vi "FPGA-7842R-Control V1.vi"(0 "Waveform Data":T4, 2 "Action":T5=enum."Exit", 3 "Laser On Time (Ticks)":u8=13, 5 "Laser Controls":T1 {"STED Power (V)" scale=0.0..10.0}, 7 "Manual Controls":T3={"Galvo 1 Position (I16)"=-280, "Galvo 2 Position (I16)"=-280, "X Axis Voltage (I16)"=0, "Y Axis Voltage (I16)"=0, "Z Axis Voltage (I16)"=0, "Res Mirror Amp (I16)"=0, "Res Mirror Mute"=FALSE, "Upper Shutter"=FALSE, "Lower Shutter"=FALSE}, 9 "Image Acquisition Parameters":T2={"Scan Type"=enum."Sample Scanning", "Scan Mode"=enum."XY", "Fast Axis Frequency (Hz)"=100.0, "Image Format"=128, "Line Accumulations"=1, "Frames Per Capture"=1, "Frames Accumulations"=1, "Image Dimension (um)"=[], "Number of Z Steps"=1, "Z Steps Size (um)"=1.0, "Pixel Size (nm)"=[]} {"Z Steps Size (um)" min=0.0; "Number of Z Steps" min=1; "Frames Accumulations" min=1; "Frames Per Capture" min=1; "Line Accumulations" min=1; "Image Format" items=["64 x 64"=64, "128 x 128"=128, "256 x 256"=256, "512 x 512"=512, "1024 x 1024"=1024, "2048 x 2048"=2048]}, 11 "Initialize":bool, 12 "Unused Axis Offset (I16)":i16, 14 "Laser Delay (Ticks)":u8=6) -> (4 "Shutter Status":cluster{"US Status":bool, "LS Status":bool}, 15 "Initalized":bool)   [LabVIEW 2014]
uses:
  FPGA-7842R-Reference.ctl
  Waveform Data.ctl
  Manual Controls V2.ctl
  Type Defs/Image Acquisition Parameters.ctl
  Laser Controls.ctl
  <vilib>/FPGAPlugInAG/PCIe-7841R/niLvFpga_Open_PCIe-7841R.vi
  <vilib>/Utility/error.llb/Error Cluster From Error Code.vi
  <vilib>/rvi/errors/niLvFpgaAdjustHostInterfaceError.vi
  <vilib>/FPGAPlugInAG/PCIe-7841R/niLvFpga_Run_PCIe-7841R.vi
  <vilib>/FPGAPlugInAG/PCIe-7841R/niLvFpga_Close_PCIe-7841R.vi
  <vilib>/rvi/interface/nirviOpenFPGA/nirviOpenFPGA.xnode
  FPGA Bitfiles/MainSTEDFPGAProj_FPGATarget_WaveformandLaser_ZYWKw02D2jI.lvbitx
  FPGA Target VIs/FPGA-7841R/Waveform and Laser Controls V5.vi
  <vilib>/rvi/interface/nirviReadWriteControl/nirviReadWriteControl.xnode
  FPGA Target VIs/FPGA-7841R/Waveform Scan Parameters.ctl
  <vilib>/rvi/interface/nirviMethod/nirviMethod.xnode
  <vilib>/rvi/interface/nirviCloseFPGA/nirviCloseFPGA.xnode
  NiFpgaLv.dll
panel:
  # "XY"
  # "Z"
  # "Length"
  # "Height"
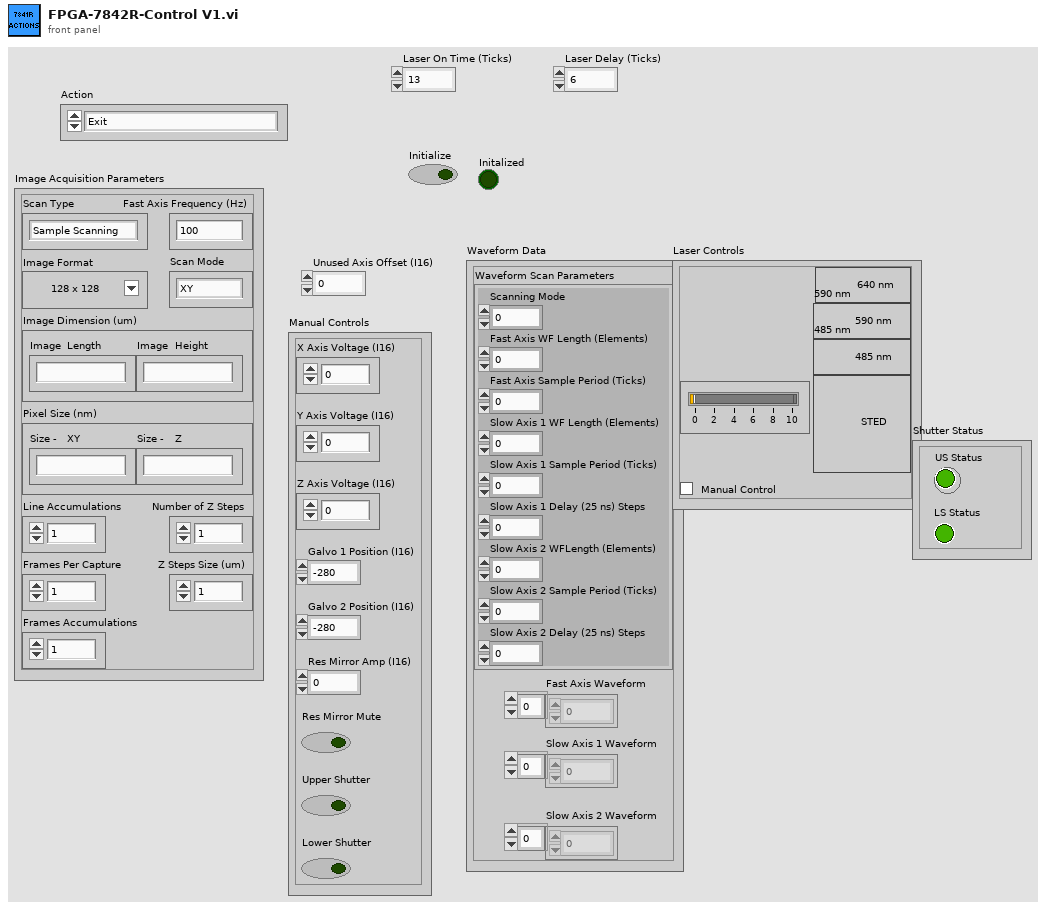
[diagram p1: front panel]
types:
  T1 = typedef "Laser Controls.ctl" = cluster{"STED Power (V)":dbl, "STED":bool, "650 nm":bool, "590 nm":bool, "485 nm":bool, "Manual Control":bool}
  T2 = typedef "Image Acquisition Parameters.ctl" = cluster{"Scan Type":enum16{"Sample Scanning", "Beam Scanning"}, "Scan Mode":enum16{"XY", "XZ", "YZ", "XYZ"}, "Fast Axis Frequency (Hz)":dbl, "Image Format":u16, "Line Accumulations":u16, "Frames Per Capture":u16, "Frames Accumulations":u16, "Image Dimension (um)":dbl[], "Number of Z Steps":u8, "Z Steps Size (um)":dbl, "Pixel Size (nm)":dbl[]}
  T3 = typedef "Manual Controls V2.ctl" = cluster{"Galvo 1 Position (I16)":i16, "Galvo 2 Position (I16)":i16, "X Axis Voltage (I16)":i16, "Y Axis Voltage (I16)":i16, "Z Axis Voltage (I16)":i16, "Res Mirror Amp (I16)":i16, "Res Mirror Mute":bool, "Upper Shutter":bool, "Lower Shutter":bool}
  T4 = typedef "Waveform Data.ctl" = cluster{"Waveform Scan Parameters":cluster{"Scanning Mode":u8, "Fast Axis WF Length (Elements)":i32, "Fast Axis Sample Period (Ticks)":u32, "Slow Axis 1 WF Length (Elements)":i32, "Slow Axis 1 Sample Period (Ticks)":u32, "Slow Axis 1 Delay (25 ns) Steps":i32, "Slow Axis 2 WFLength (Elements)":i32, "Slow Axis 2 Sample Period (Ticks)":u32, "Slow Axis 2 Delay (25 ns) Steps":i32}, "Fast Axis Waveform":dbl[], "Slow Axis 1 Waveform":dbl[], "Slow Axis 2 Waveform":dbl[]}
  T5 = typedef "FPGA-7842R-Reference.ctl" = enum16{"Stage Control", "Laser Control", "Unused Axis I16", "Exit", "Set Res Mirror", "Set Galvo", "Current Frame for Capture", "Default", "Close FPGA", "Stop Waveforms", "Start Waveforms", "Shutter Control", "Initialize"}
  T6 = cluster{"Scanning Mode":u8, "Fast Axis WF Length (Elements)":i32, "Fast Axis Sample Period (Ticks)":u32, "Slow Axis 1 WF Length (Elements)":i32, "Slow Axis 1 Sample Period (Ticks)":u32, "Slow Axis 1 Delay (25 ns) Steps":i32, "Slow Axis 2 WFLength (Elements)":i32, "Slow Axis 2 Sample Period (Ticks)":u32, "Slow Axis 2 Delay (25 ns) Steps":i32}
  T7 = cluster{"Res Mirror Amp (I16)":i16, "Res Mirror Mute":bool}
  T8 = typedef "Scan Parameters.ctl" = cluster{"Fast_Ax_Amp_V":dbl, "Fast_Ax_Off_V":dbl, "Slow_Ax_Amp_V":dbl, "Slow_Ax_Off_V ":dbl, "Slow_Ax_Max_V_VperS":dbl, "Slow_Ax1_Del25ns":i32, "Slow_Ax2_Del25ns":i32, "Stage_X_Off_V":dbl, "Stage_Y_Off_V":dbl, "Stage_Z_Off_V":dbl, "Galvo1_Off_V":dbl, "Galvo2_Off_V":dbl, "Last_Scan_Mode":enum16{"XY", "XZ", "YZ", "XYZ"}, "Current_Scan_Mode":enum16{"XY", "XZ", "YZ", "XYZ"}, "Fly_Back_Lines":u16, "Linear_Ramp_End":u32, "Z_Step_I16":i16, "Z_Start_I16":i16, "Laser_States _U32":u32, "590_Voltage_I16":i16, "775_AOM_Volt_I16":i16, "Blanking OFF":bool, "Unused_Axis_I16":i16}
  T9 = cluster{"Upper Shutter Status":bool, "Lower Shutter Status":bool}
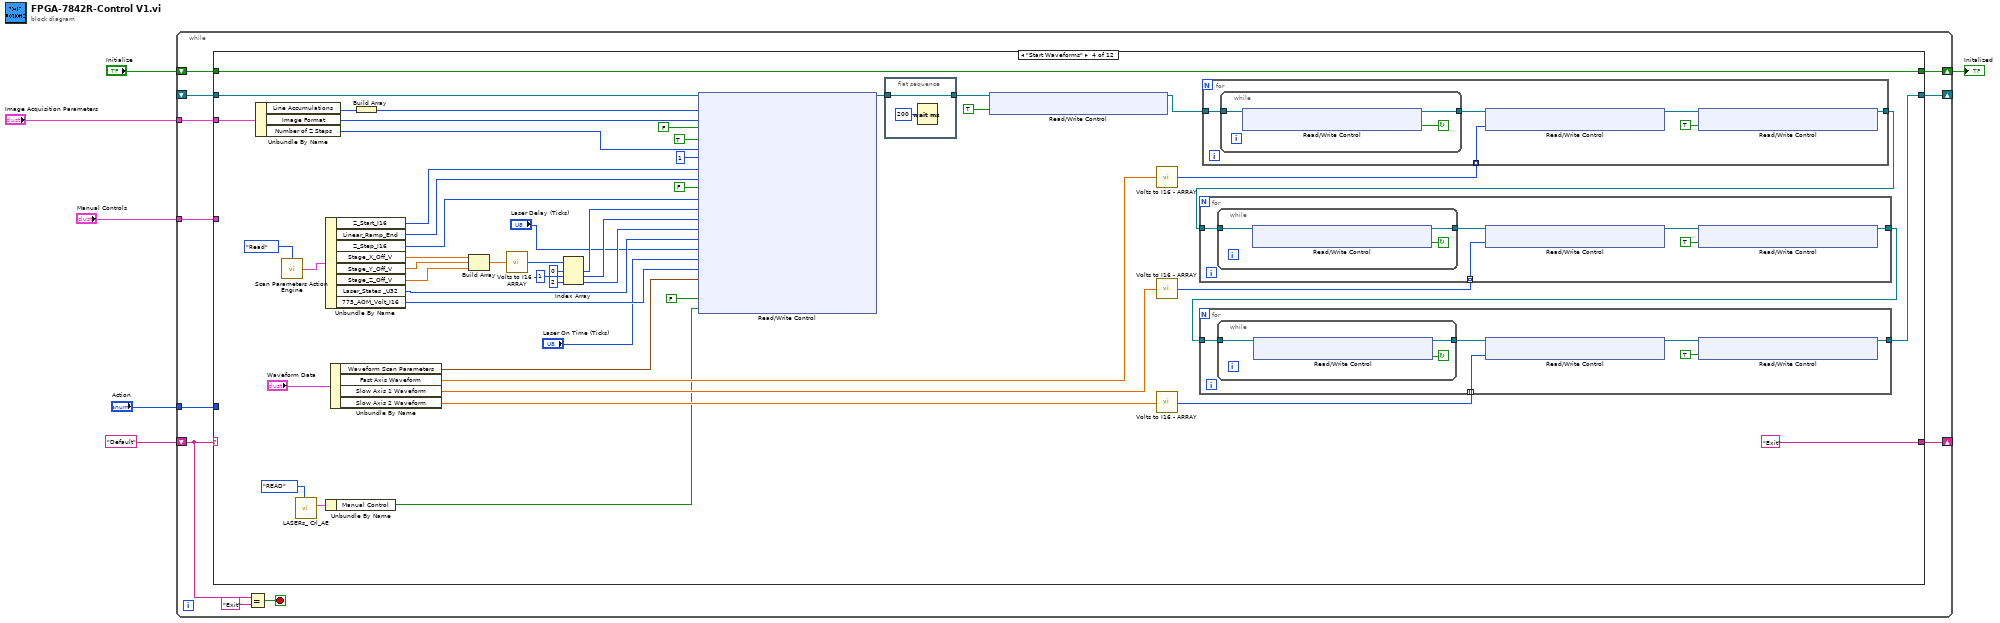
[diagram p0: block diagram]
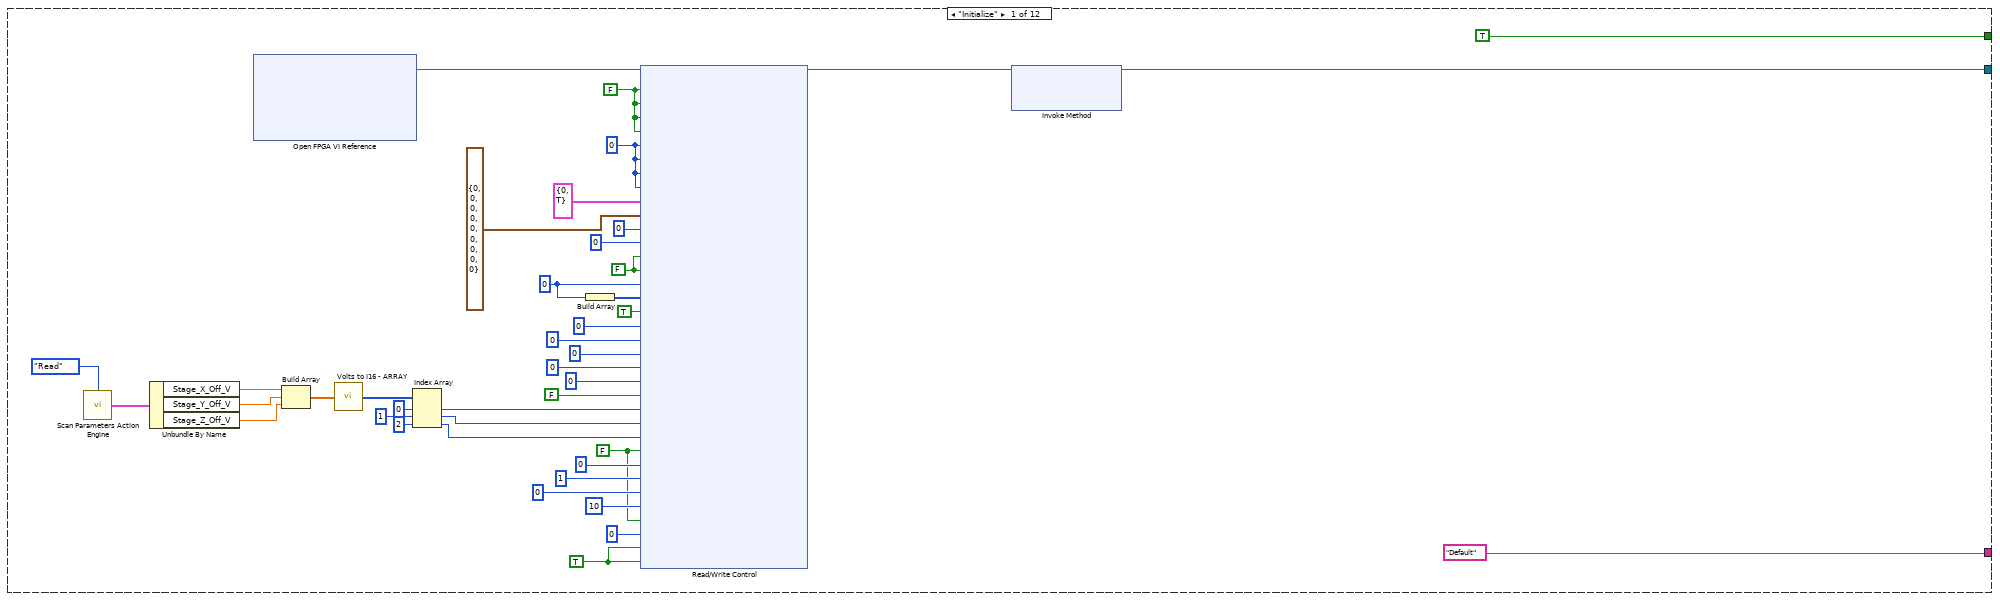
[diagram p2: hidden frame]
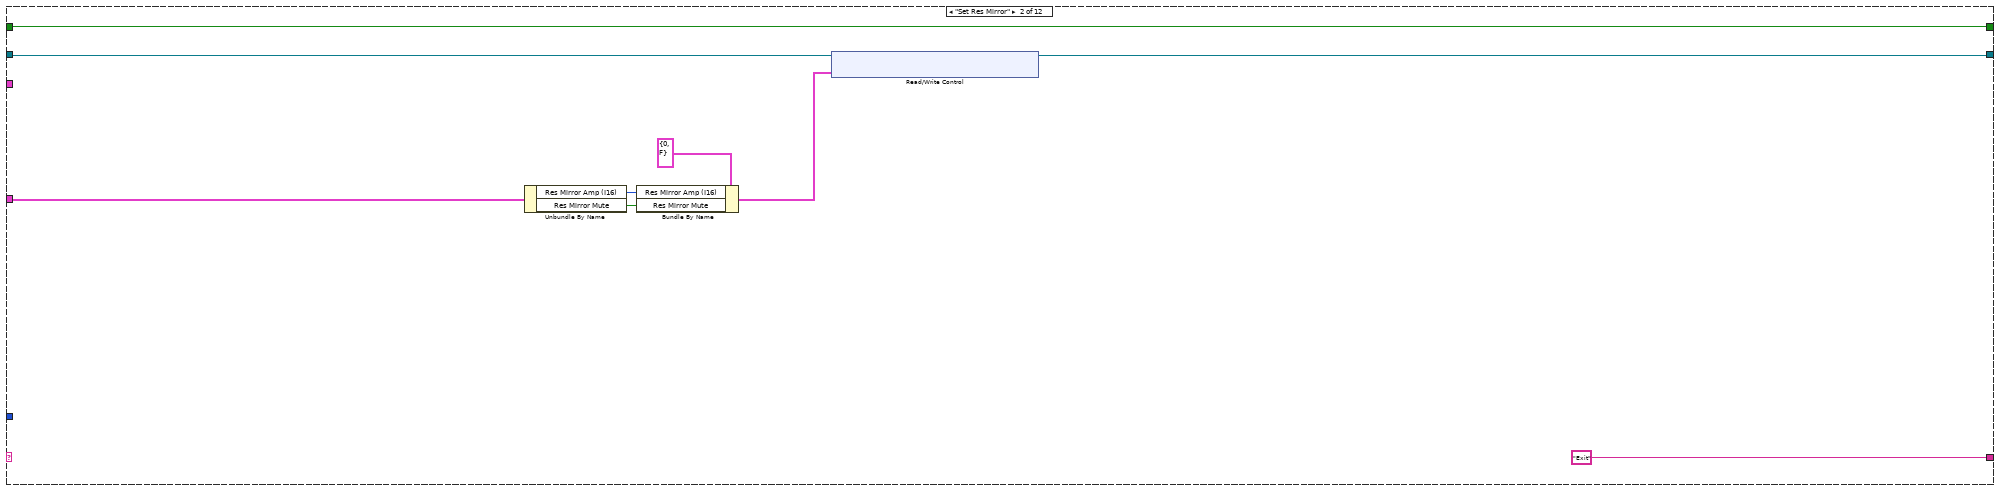
[diagram p3: hidden frame]
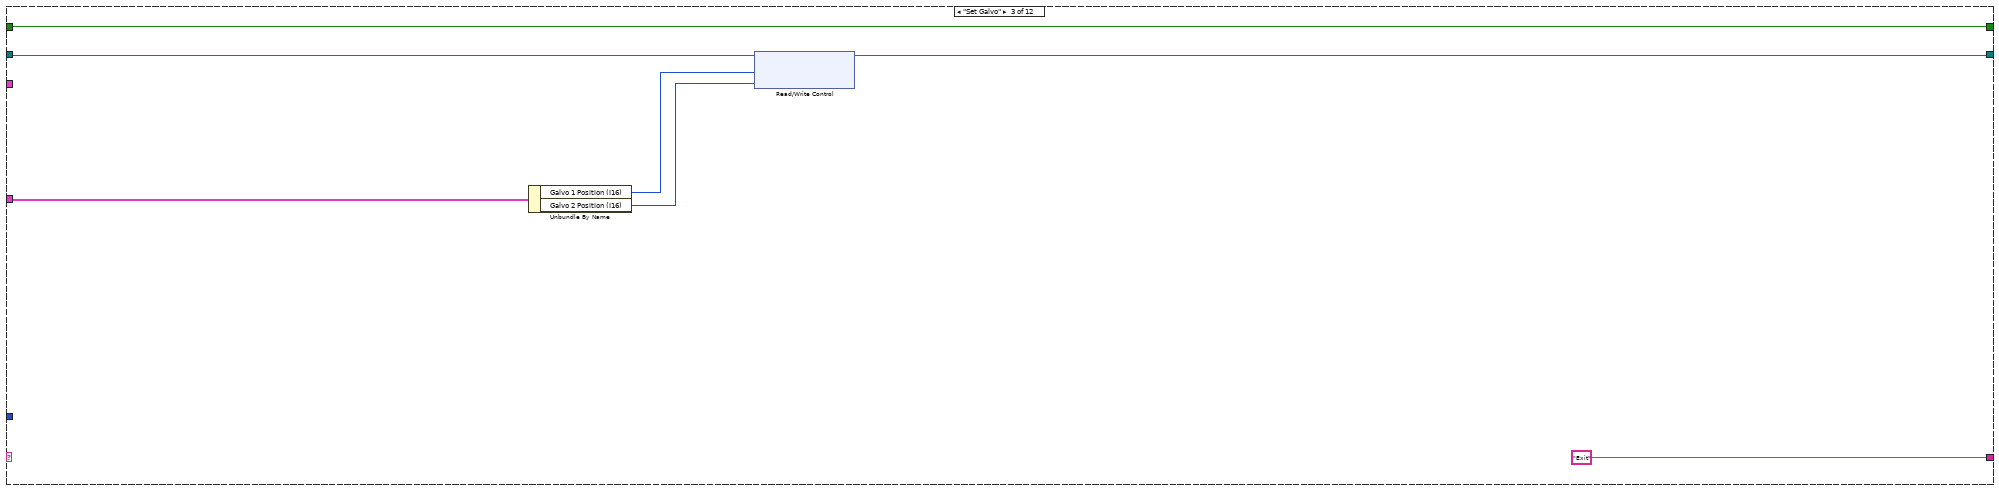
[diagram p4: hidden frame]
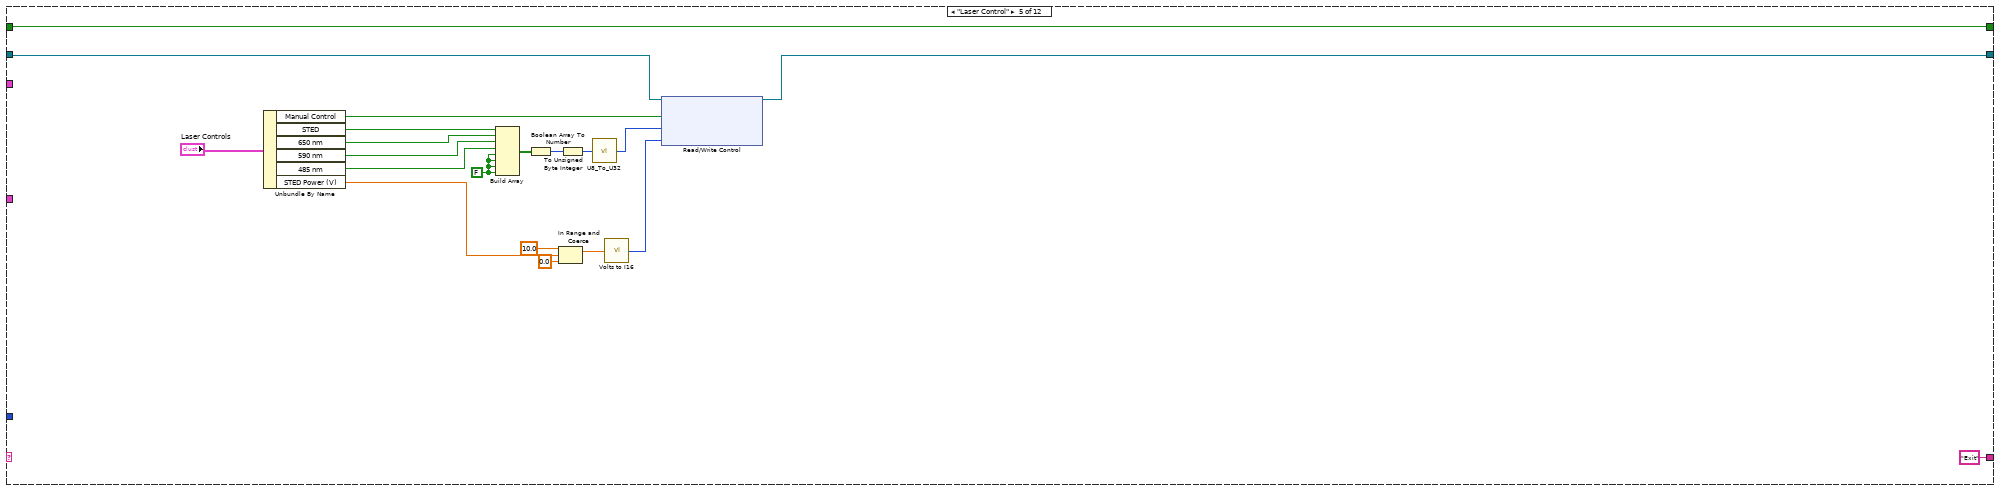
[diagram p5: hidden frame]
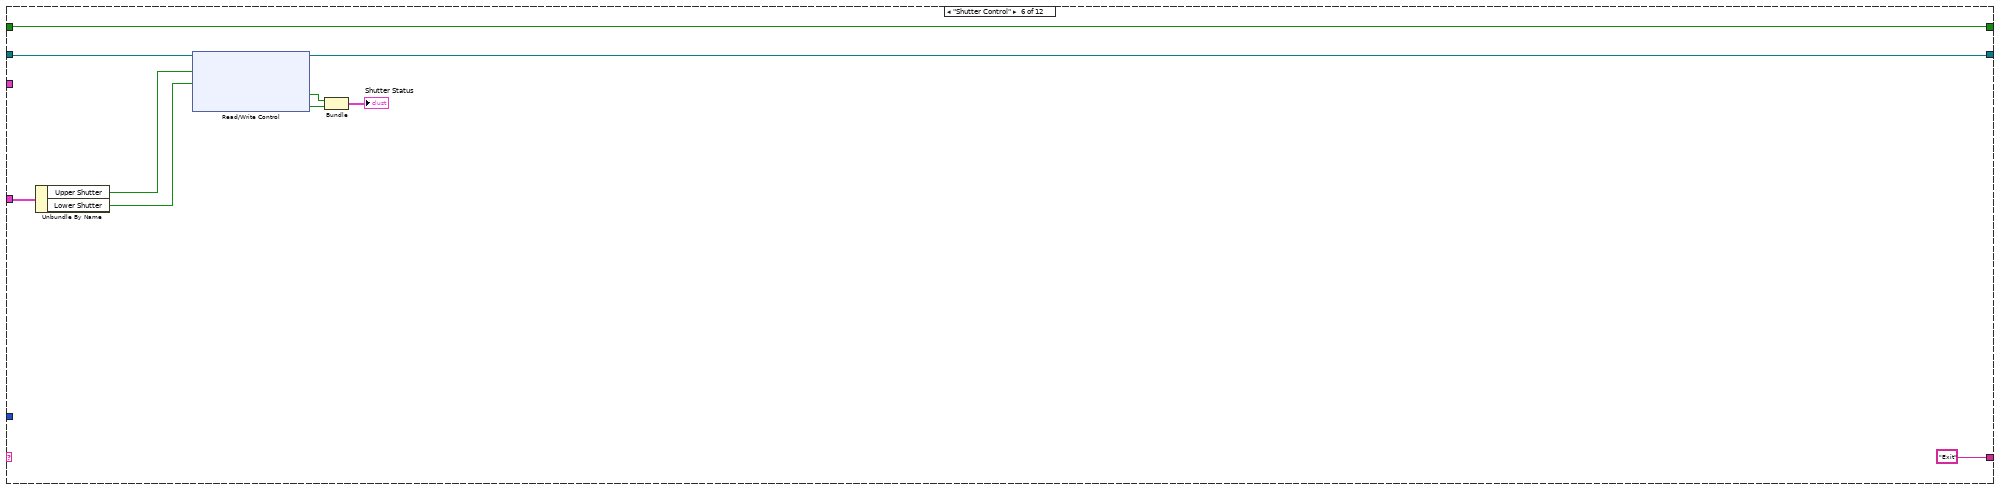
[diagram p6: hidden frame]
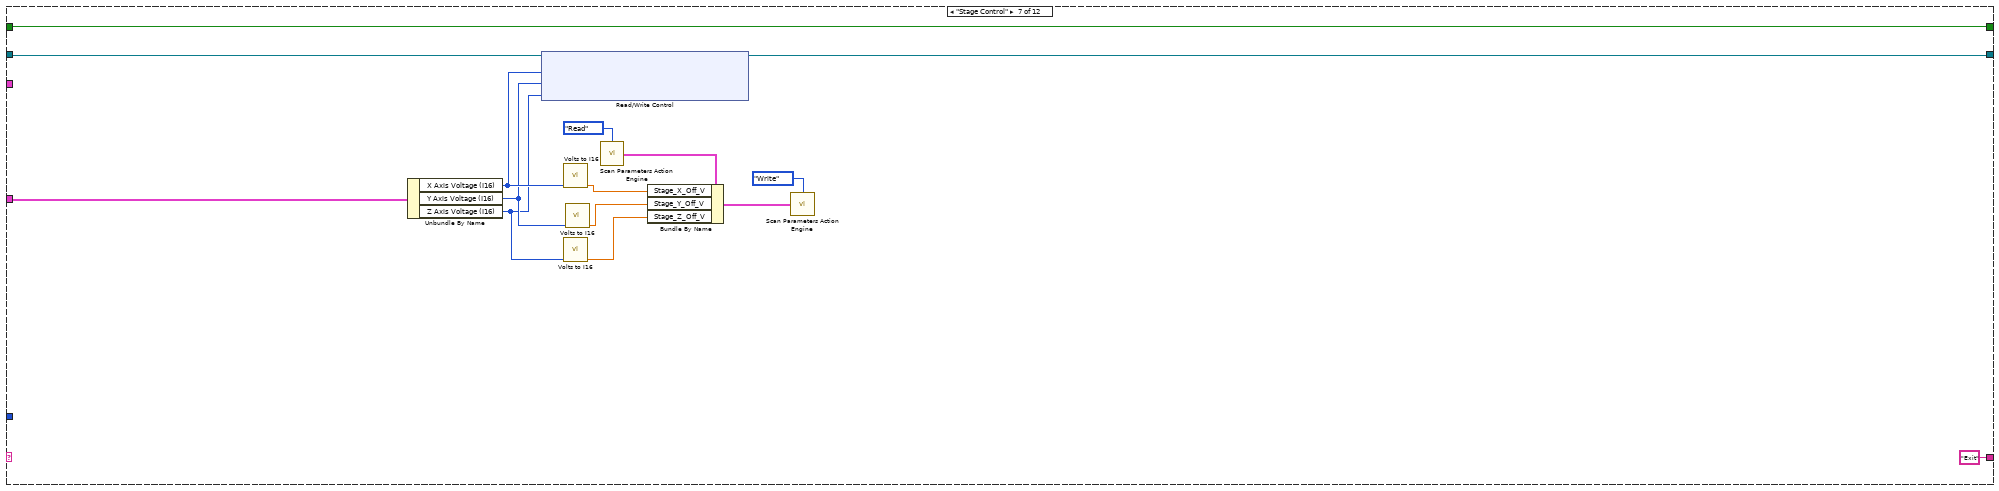
[diagram p7: hidden frame]
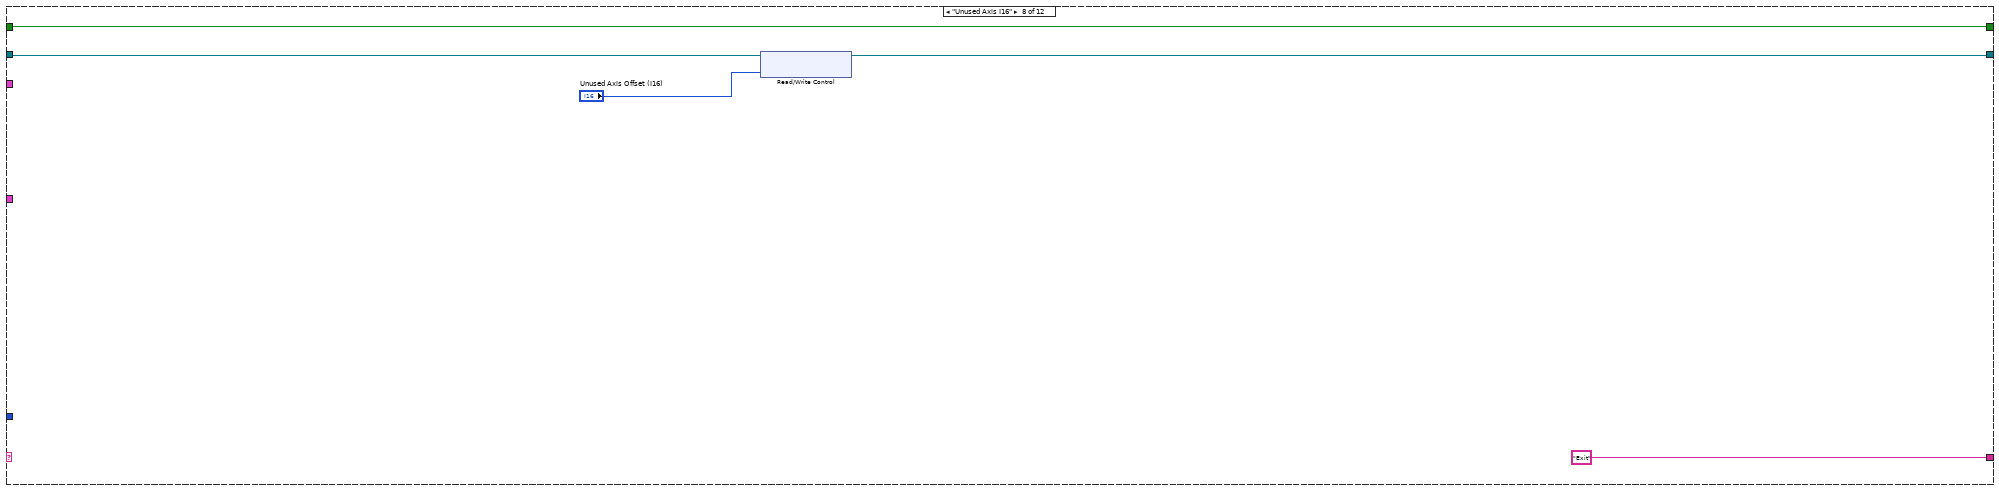
[diagram p8: hidden frame]
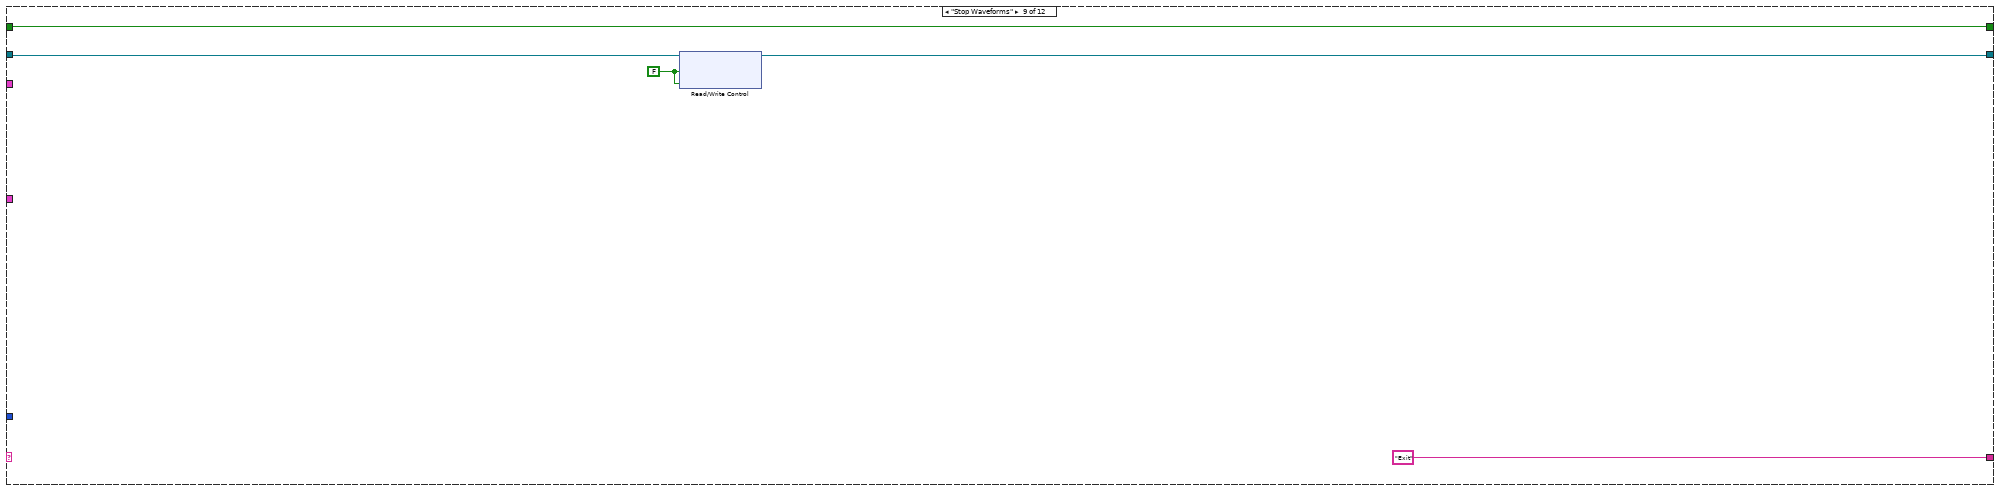
[diagram p9: hidden frame]
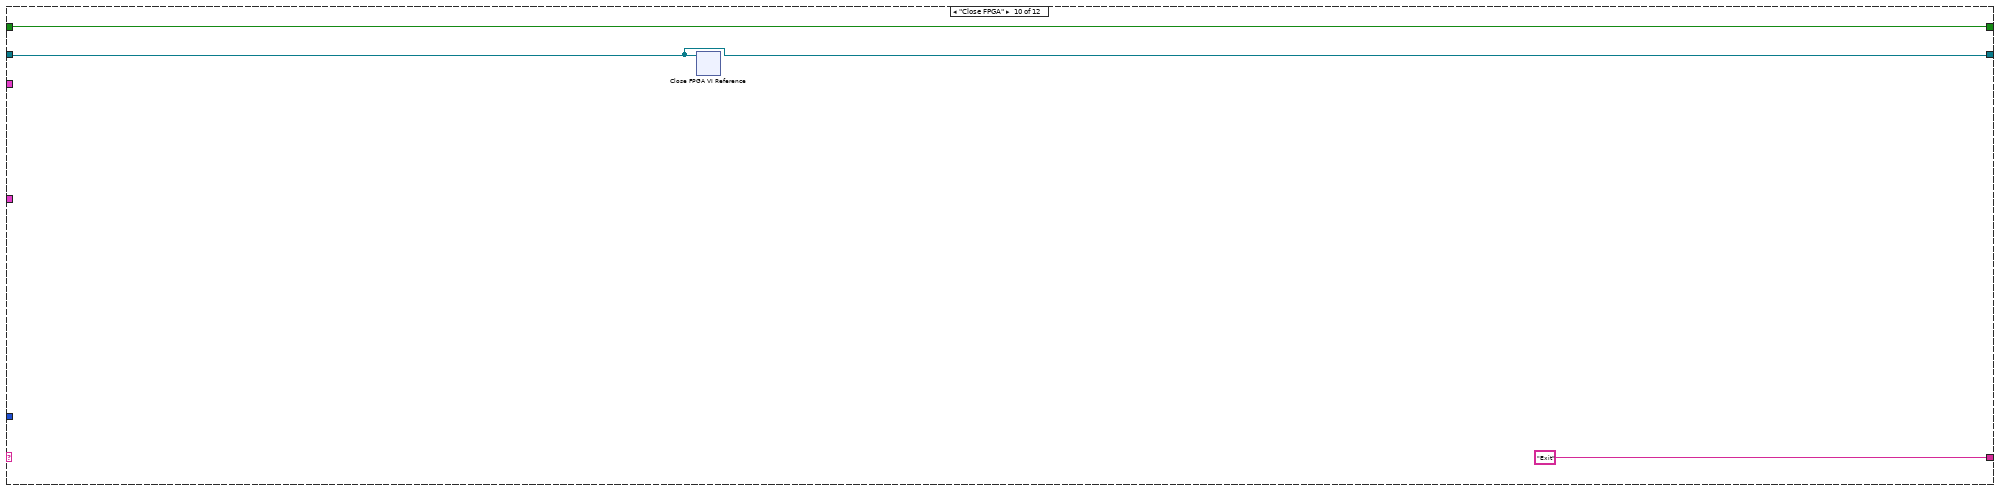
[diagram p10: hidden frame]
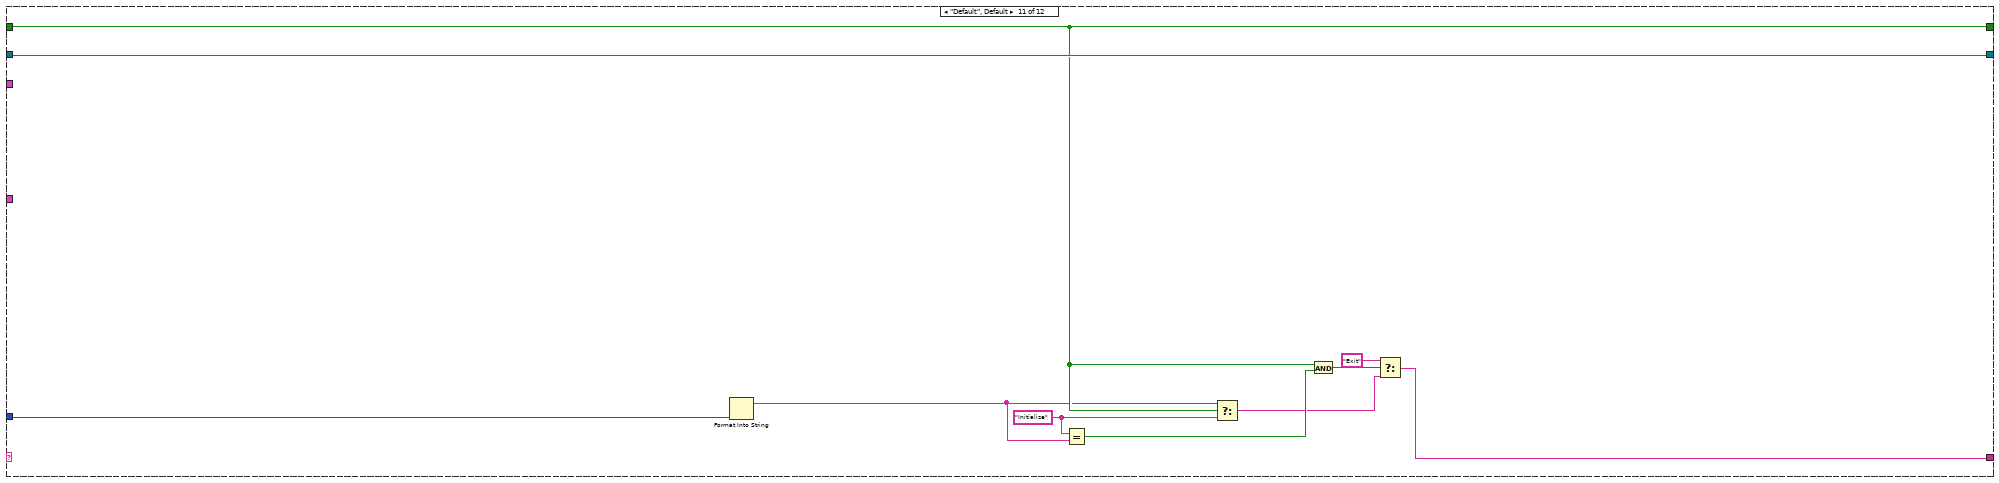
[diagram p11: hidden frame]
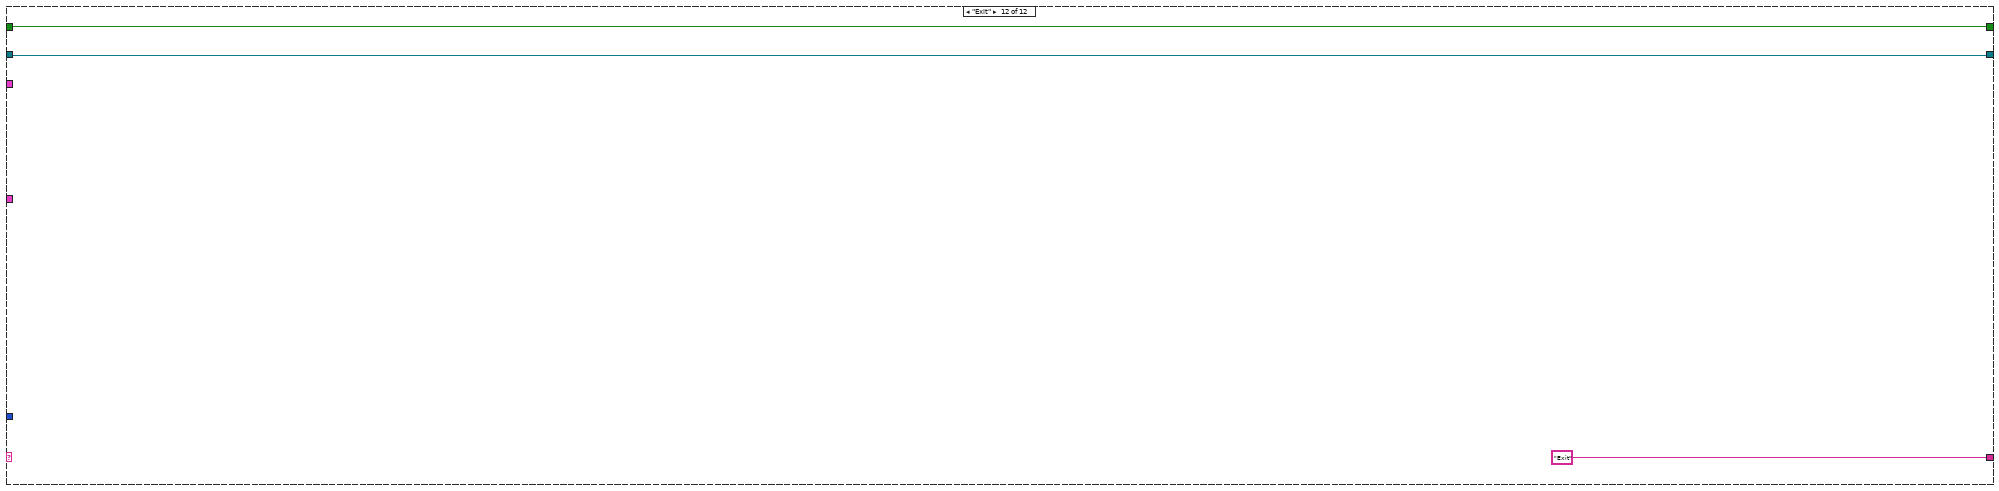
[diagram p12: hidden frame]
diagram:
  n1 = while {
    shift-right: [w17] -> _
    shift-left: _ -> [w16]
    shift-right: [w14] -> _
    shift-left: "Default" -> [w13]
    tunnel: "Action" -> [w15]
    shift-right: [w10] -> w3
    shift-left: "Initialize" -> [w9]
    tunnel: "Manual Controls" -> [w8]
    tunnel: "Image Acquisition Parameters" -> [w7]
    stop <- w11 stop-if-true
    n2 = case shown="\"Start Waveforms\"" w13 {
      tunnel: [w49 w64 w71 w114 w170 w182 w195 w201 w208 w210 w222 w224] -> w17
      tunnel: w16 -> [_ w65 w72 w117 w171 w183 w196 w202 w209 w210 w222 w224]
      tunnel: w15 -> [_ _ _ _ _ _ _ _ _ _ w221 _]
      tunnel: ["Default" ("f") "Exit" ("f") "Exit" ("f") "Exit" ("f") "Exit" ("f") "Exit" ("f") "Exit" ("f") "Exit" ("f") "Exit" ("f") "Exit" ("f") w215 "Exit" ("f")] -> w14
      tunnel: [TRUE w67 w74 w119 w173 w184 w198 w204 w207 w212 w220 w225] -> w10
      tunnel: w9 -> [_ w67 w74 w119 w173 w184 w198 w204 w207 w212 w220 w225]
      tunnel: w8 -> [_ w63 w70 _ _ w177 w197 _ _ _ _ _]
      tunnel: w7 -> [_ _ _ w108 _ _ _ _ _ _ _ _]
      frame "Initialize" {
        w18 = TRUE ("Upper Shutter Command")
        w20 = FALSE ("Blanking Off/Manual")
        w45 = u16 0 ("Number of Lines")
        w47 = FALSE ("Reset Position Error")
        w58 = i16 0 ("Fast Axis Waveform Element")
        w57 = FALSE ("WF 1 Data Loaded")
        n3 = call "Scan Parameters Action Engine.vi"("Action"=enum16{"Read", "Write"}."Read") -> ("Scan Parameters OUT"=w36:T8)  [unwired: 14 in]
        n4 = Unbundle By Name(w36) -> ("Stage_X_Off_V"=w35:dbl, "Stage_Y_Off_V"=w33:dbl, "Stage_Z_Off_V"=w34:dbl)
        n5 = xnode "Open FPGA VI Reference"() -> ("FPGA VI Reference Out"=w48:refnum<k20>)  [unwired: 2 in, 1 out]
        n6 = Build Array(w35, w33, w34) -> (w32:dbl[])
        n7 = call "Volts to I16 - ARRAY.vi"("Voltage (V)"=w32) -> ("I16"=w31:i16[])  [unwired: 14 in]
        n8 = Index Array(array=w31, index #1=0 ("index"), index #2=1 ("index"), index #3=2 ("index")) -> (element #1=w27:i16, element #2=w25:i16, element #3=w26:i16)
        n9 = Build Array(w45) -> (w44:u16[])
        n10 = xnode "Read/Write Control"("FPGA VI Reference In"=w48, "WF 1 Data Loaded"=w57, "WF 2 Data Loaded"=w57, "WF 3 Data Loaded"=w57, "Start Waveforms"=w57, "Fast Axis Waveform Element"=w58, "Slow Axis 1 Waveform Element"=w58, "Slow Axis 2 Waveform Element"=w58, "Unused Axis Offset"=w58, "Resonant Mirror"=T7 {"Res Mirror Amp (I16)"=0, "Res Mirror Mute"=TRUE} ("Resoance Mirror"), "Waveform Scan Parameters"=T6 {"Scanning Mode"=0, "Fast Axis WF Length (Elements)"=0, "Fast Axis Sample Period (Ticks)"=0, "Slow Axis 1 WF Length (Elements)"=0, "Slow Axis 1 Sample Period (Ticks)"=0, "Slow Axis 1 Delay (25 ns) Steps"=0, "Slow Axis 2 WFLength (Elements)"=0, "Slow Axis 2 Sample Period (Ticks)"=0, "Slow Axis 2 Delay (25 ns) Steps"=0}, "Galvo 2 Position (I16)"=i16 0, "Galvo 1 Position (I16)"=i16 0, "Reset Position Error"=w47, "Frame Trigger"=w47, "Number of Lines"=w45, "Accums Per Line"=w44, "Stop Sync Signal"=TRUE, "Z Step Size (I16)"=i16 0, "Number of Z Steps"=u8 0, "Frames Per Z Step"=u8 0, "Z Stack Start Position (I16)"=i16 0, "End of Linear Ramp"=u32 0, "End Linear Ramp"=FALSE, "X Piezo Axis"=w27, "Y Piezo Axis"=w25, "Z Piezo Axis"=w26, "Blanking Off/Manual"=w20, "Laser States"=u32 0, "Laser Delay (Ticks)"=u8 1, "Sequences"=u8 0, "Laser On Time (Ticks)"=u8 10, "Laser Blank Trigger"=w20, "775 AOM (I16)"=i16 0 ("590 Analog Voltage (I16)"), "Upper Shutter Command"=w18, "Lower Shutter Command"=w18) -> ("FPGA VI Reference Out"=w54:refnum<k20>)  [unwired: 1 in, 1 out]
        n11 = xnode "Invoke Method"("FPGA VI Reference In"=w54) -> ("FPGA VI Reference Out"=w49:refnum<k20>)  [unwired: 2 in, 1 out]
      }
      frame "Set Res Mirror" {
        n12 = Unbundle By Name(w63) -> ("Res Mirror Amp (I16)"=w62:i16, "Res Mirror Mute"=w61:bool)
        n13 = Bundle By Name(cluster=T7 {"Res Mirror Amp (I16)"=0, "Res Mirror Mute"=FALSE} ("Resoance Mirror"), "Res Mirror Amp (I16)"=w62, "Res Mirror Mute"=w61) -> (w59:T7)
        n14 = xnode "Read/Write Control"("FPGA VI Reference In"=w65, "Resonant Mirror"=w59) -> ("FPGA VI Reference Out"=w64:refnum<k20>)  [unwired: 1 in, 1 out]
      }
      frame "Set Galvo" {
        n15 = Unbundle By Name(w70) -> ("Galvo 1 Position (I16)"=w69:i16, "Galvo 2 Position (I16)"=w68:i16)
        n16 = xnode "Read/Write Control"("FPGA VI Reference In"=w72, "Galvo 1 Position (I16)"=w69, "Galvo 2 Position (I16)"=w68) -> ("FPGA VI Reference Out"=w71:refnum<k20>)  [unwired: 1 in, 1 out]
      }
      frame "Start Waveforms" {
        n17 = Unbundle By Name(w108) -> ("Line Accumulations"=w106:u16, "Image Format"=w107:u16, "Number of Z Steps"=w97:u8)
        n18 = call "Scan Parameters Action Engine.vi"("Action"=enum16{"Read", "Write"}."Read") -> ("Scan Parameters OUT"=w101:T8)  [unwired: 14 in]
        n19 = call "LASERs_ Crl_AE.vi"("Action"=enum16{"READ", "WRITE"}."READ") -> ("Detectors Parameters Out"=w76:T1)  [unwired: 10 in]
        n20 = Unbundle By Name(w101) -> ("Z_Start_I16"=w99:i16, "Linear_Ramp_End"=w100:u32, "Z_Step_I16"=w96:i16, "Stage_X_Off_V"=w89:dbl, "Stage_Y_Off_V"=w88:dbl, "Stage_Z_Off_V"=w87:dbl, "Laser_States _U32"=w83:u32, "775_AOM_Volt_I16"=w82:i16)
        n21 = Unbundle By Name(w76) -> ("Manual Control"=w75:bool)
        n22 = Unbundle By Name("Waveform Data") -> ("Waveform Scan Parameters"=w81:T6, "Fast Axis Waveform"=w121:dbl[], "Slow Axis 1 Waveform"=w113:dbl[], "Slow Axis 2 Waveform"=w120:dbl[])
        n23 = Build Array(w106) -> (w105:u16[])
        n24 = Build Array(w89, w88, w87) -> (w94:dbl[])
        n25 = call "Volts to I16 - ARRAY.vi"("Voltage (V)"=w94) -> ("I16"=w93:i16[])  [unwired: 14 in]
        n26 = Index Array(array=w93, index #1=0 ("index"), index #2=1 ("index"), index #3=2 ("index")) -> (element #1=w86:i16, element #2=w85:i16, element #3=w84:i16)
        n27 = xnode "Read/Write Control"("FPGA VI Reference In"=w117, "Accums Per Line"=w105, "Number of Lines"=w107, "Frame Trigger"=FALSE, "Stop Sync Signal"=TRUE, "Number of Z Steps"=w97, "Frames Per Z Step"=u8 1, "Z Stack Start Position (I16)"=w99, "End of Linear Ramp"=w100, "End Linear Ramp"=FALSE, "Z Step Size (I16)"=w96, "X Piezo Axis"=w86, "Y Piezo Axis"=w85, "Z Piezo Axis"=w84, "Laser States"=w83, "Laser Delay (Ticks)"="Laser Delay (Ticks)", "Laser On Time (Ticks)"="Laser On Time (Ticks)", "775 AOM (I16)"=w82, "Waveform Scan Parameters"=w81, "Frame Trigger"=FALSE, "Blanking Off/Manual"=w75) -> ("FPGA VI Reference Out"=w115:refnum<k20>)  [unwired: 1 in, 2 out]
        n28 = flat-sequence {
          tunnel: [w127] -> w116
          tunnel: w115 -> [w127]
          frame #0 {
            n29 = Wait (ms)(milliseconds to wait=u32 200) -> ()  [unwired: 1 out]
          }
        }
        n30 = xnode "Read/Write Control"("FPGA VI Reference In"=w116, "Start Waveforms"=TRUE) -> ("FPGA VI Reference Out"=w122:refnum<k20>)  [unwired: 1 in, 1 out]
        n31 = call "Volts to I16 - ARRAY.vi"("Voltage (V)"=w121) -> ("I16"=w125:i16[])  [unwired: 14 in]
        n32 = call "Volts to I16 - ARRAY.vi"("Voltage (V)"=w113) -> ("I16"=w111:i16[])  [unwired: 14 in]
        n33 = call "Volts to I16 - ARRAY.vi"("Voltage (V)"=w120) -> ("I16"=w112:i16[])  [unwired: 14 in]
        n34 = for {
          tunnel: w122 -> [w150]
          tunnel: [w148] -> w124
          tunnel: w125 -> [w146] mode=indexing
          n35 = while {
            tunnel: w150 -> [w154]
            tunnel: [w153] -> w149
            stop <- w152 continue-if-true
            n36 = xnode "Read/Write Control"("FPGA VI Reference In"=w154) -> ("FPGA VI Reference Out"=w153:refnum<k20>, "WF 1 Data Loaded"=w152:bool)  [unwired: 1 in, 1 out]
          }
          n37 = xnode "Read/Write Control"("FPGA VI Reference In"=w149, "Fast Axis Waveform Element"=w146) -> ("FPGA VI Reference Out"=w151:refnum<k20>)  [unwired: 1 in, 1 out]
          n38 = xnode "Read/Write Control"("FPGA VI Reference In"=w151, "WF 1 Data Loaded"=TRUE ("Host Data Loaded")) -> ("FPGA VI Reference Out"=w148:refnum<k20>)  [unwired: 1 in, 1 out]
        }
        n39 = for {
          tunnel: w124 -> [w141]
          tunnel: [w139] -> w95
          tunnel: w111 -> [w137] mode=indexing
          n40 = while {
            tunnel: w141 -> [w145]
            tunnel: [w144] -> w140
            stop <- w143 continue-if-true
            n41 = xnode "Read/Write Control"("FPGA VI Reference In"=w145) -> ("FPGA VI Reference Out"=w144:refnum<k20>, "WF 2 Data Loaded"=w143:bool)  [unwired: 1 in, 1 out]
          }
          n42 = xnode "Read/Write Control"("FPGA VI Reference In"=w140, "Slow Axis 1 Waveform Element"=w137) -> ("FPGA VI Reference Out"=w142:refnum<k20>)  [unwired: 1 in, 1 out]
          n43 = xnode "Read/Write Control"("FPGA VI Reference In"=w142, "WF 2 Data Loaded"=TRUE ("Host Data Loaded")) -> ("FPGA VI Reference Out"=w139:refnum<k20>)  [unwired: 1 in, 1 out]
        }
        n44 = for {
          tunnel: w95 -> [w132]
          tunnel: [w130] -> w114
          tunnel: w112 -> [w128] mode=indexing
          n45 = while {
            tunnel: w132 -> [w136]
            tunnel: [w135] -> w131
            stop <- w134 continue-if-true
            n46 = xnode "Read/Write Control"("FPGA VI Reference In"=w136) -> ("FPGA VI Reference Out"=w135:refnum<k20>, "WF 3 Data Loaded"=w134:bool)  [unwired: 1 in, 1 out]
          }
          n47 = xnode "Read/Write Control"("FPGA VI Reference In"=w131, "Slow Axis 2 Waveform Element"=w128) -> ("FPGA VI Reference Out"=w133:refnum<k20>)  [unwired: 1 in, 1 out]
          n48 = xnode "Read/Write Control"("FPGA VI Reference In"=w133, "WF 3 Data Loaded"=TRUE ("Host Data Loaded")) -> ("FPGA VI Reference Out"=w130:refnum<k20>)  [unwired: 1 in, 1 out]
        }
      }
      frame "Laser Control" {
        w164 = FALSE ("element")
        n49 = Unbundle By Name("Laser Controls") -> ("Manual Control"=w172:bool, "STED"=w161:bool, "650 nm"=w160:bool, "590 nm"=w159:bool, "485 nm"=w158:bool, "STED Power (V)"=w157:dbl)
        n50 = Build Array(w161, w160, w159, w158, w164, w164, w164, w164) -> (w162:bool[])
        n51 = Boolean Array To Number(Boolean array=w162) -> (number=w163:u32)
        n52 = In Range and Coerce(upper limit=10.0, x=w157, lower limit=0.0) -> (coerced(x)=w168:dbl)  [unwired: 1 out]
        n53 = To Unsigned Byte Integer(number=w163) -> (unsigned 8bit integer=w165:u8)
        n54 = call "U8_To_U32.vi"("U8 IN"=w165) -> ("U32 OUT"=w156:u32)  [unwired: 13 in, 1 out]
        n55 = call "Volts to I16.vi"("Voltage (V)"=w168) -> ("I16"=w155:i16)  [unwired: 13 in, 1 out]
        n56 = xnode "Read/Write Control"("FPGA VI Reference In"=w171, "Blanking Off/Manual"=w172, "Laser States"=w156, "775 AOM (I16)"=w155) -> ("FPGA VI Reference Out"=w170:refnum<k20>)  [unwired: 1 in, 1 out]
      }
      frame "Shutter Control" {
        n57 = Unbundle By Name(w177) -> ("Upper Shutter"=w175:bool, "Lower Shutter"=w176:bool)
        n58 = xnode "Read/Write Control"("FPGA VI Reference In"=w183, "Upper Shutter Command"=w175, "Lower Shutter Command"=w176) -> ("FPGA VI Reference Out"=w182:refnum<k20>, "Upper Shutter Status"=w180:bool, "Lower Shutter Status"=w179:bool)  [unwired: 1 in, 1 out]
        n59 = Bundle("Upper Shutter Status"=w180, "Lower Shutter Status"=w179) -> (→"Shutter Status":T9)  [unwired: 1 in]
      }
      frame "Stage Control" {
        n60 = Unbundle By Name(w197) -> ("X Axis Voltage (I16)"=w192:i16, "Y Axis Voltage (I16)"=w188:i16, "Z Axis Voltage (I16)"=w187:i16)
        n61 = xnode "Read/Write Control"("FPGA VI Reference In"=w196, "X Piezo Axis"=w192, "Y Piezo Axis"=w188, "Z Piezo Axis"=w187) -> ("FPGA VI Reference Out"=w195:refnum<k20>)  [unwired: 1 in, 1 out]
        n62 = call "Volts to I16.vi"("Volatge (I16)"=w192) -> ("Voltage (V)"=w191:dbl)  [unwired: 13 in, 1 out]
        n63 = call "Volts to I16.vi"("Volatge (I16)"=w187) -> ("Voltage (V)"=w189:dbl)  [unwired: 13 in, 1 out]
        n64 = call "Volts to I16.vi"("Volatge (I16)"=w188) -> ("Voltage (V)"=w190:dbl)  [unwired: 13 in, 1 out]
        n65 = call "Scan Parameters Action Engine.vi"("Action"=enum16{"Read", "Write"}."Read") -> ("Scan Parameters OUT"=w193:T8)  [unwired: 14 in]
        n66 = Bundle By Name(cluster=w193, "Stage_X_Off_V"=w191, "Stage_Y_Off_V"=w190, "Stage_Z_Off_V"=w189) -> (w185:T8)
        n67 = call "Scan Parameters Action Engine.vi"("Action"=enum16{"Read", "Write"}."Write", "Scan Parameters IN"=w185) -> ()  [unwired: 13 in, 1 out]
      }
      frame "Unused Axis I16" {
        n68 = xnode "Read/Write Control"("FPGA VI Reference In"=w202, "Unused Axis Offset"="Unused Axis Offset (I16)") -> ("FPGA VI Reference Out"=w201:refnum<k20>)  [unwired: 1 in, 1 out]
      }
      frame "Stop Waveforms" {
        w205 = FALSE ("Start Waveforms")
        n69 = xnode "Read/Write Control"("FPGA VI Reference In"=w209, "Start Waveforms"=w205, "Stop Sync Signal"=w205) -> ("FPGA VI Reference Out"=w208:refnum<k20>)  [unwired: 1 in, 1 out]
      }
      frame "Close FPGA" {
        n70 = xnode "Close FPGA VI Reference"("FPGA VI Reference In"=w210) -> ()  [unwired: 1 in, 1 out]
      }
      frame "Default", Default {
        w214 = "Initialize" ("f")
        n71 = Format Into String(w221) -> (resulting string=w213:string)  [unwired: 3 in, 1 out]
        n72 = Equal?(x=w214, y=w213) -> (x = y?=w219:bool)
        n73 = Select(t=w213, s=w220, f=w214) -> (s? t:f=w216:string)
        n74 = And(x=w220, y=w219) -> (x .and. y?=w218:bool)
        n75 = Select(t="Exit" ("y"), s=w218, f=w216) -> (s? t:f=w215:string)
      }
      frame "Exit" {
      }
    }
    n76 = Equal?(x=w13, y="Exit") -> (x = y?=w11:bool)
  }
  "Initalized" <- w3
